vi "Get Contained Libraries.vi"(8 "error in":errorcluster, 10 "lib data in[]":T1[](array[typedef]), 11 "library in":refnum<vi>) -> (0 "error out":errorcluster, 3 "lib data out[]":T1[](array[typedef]))   [LabVIEW 2021, in "Converter.lvlib"]
uses:
  Converter.lvlib
  TypeDefs/Library Data.ctl
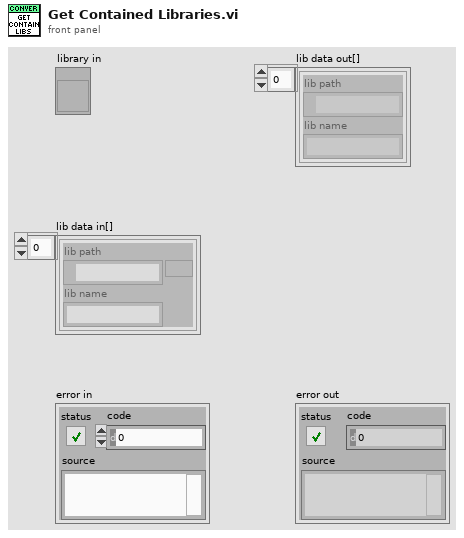
[diagram p1: front panel]
types:
  T1 = typedef "Converter.lvlib/Library Data.ctl" = cluster{"lib path":path, "lib name":string}
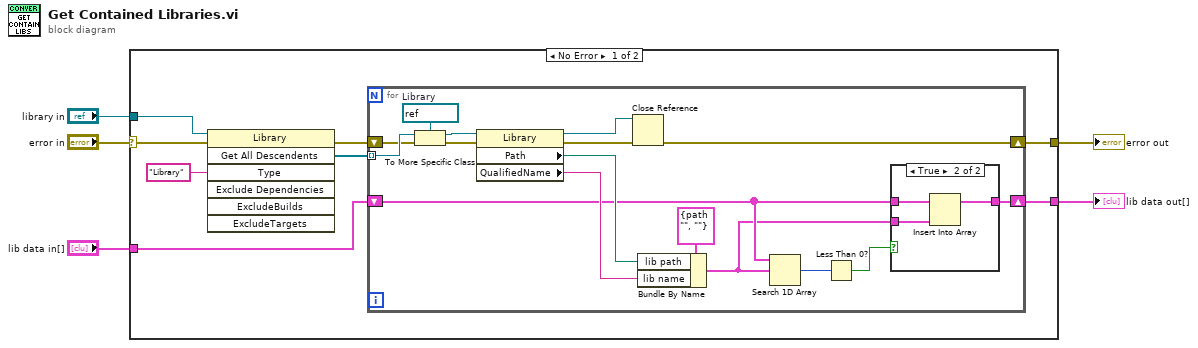
[diagram p0: block diagram]
diagram:
  n1 = case shown="No Error" "error in" {
    selector: "error in" -> [w13 w35]
    tunnel: [w6 w35] -> w5
    tunnel: "lib data in[]" -> [w12 w34]
    tunnel: [w11 w34] -> w2
    tunnel: "library in" -> [w8 _]
    frame No Error {
      n2 = invoke class="Library" method="Get All Descendents"(reference=w8, error in=w13, "Type"="Library") -> (error out=w10:errorcluster, "All Descendents"=w9:refnum<vi>[])  [unwired: 4 in, 5 out]
      n3 = for {
        tunnel: w9 -> [w29] mode=indexing
        shift-right: [w24] -> w11
        shift-left: w12 -> [w17]
        shift-right: [w14] -> w6
        shift-left: w10 -> [w27]
        w25 = refnum<vi> refnum  # Library
        n4 = To More Specific Class(target class=w25, reference=w29, error in=w27) -> (specific class reference=w28:refnum<vi>, error out=w26:errorcluster)
        n5 = property class="Library"(reference=w28, error in=w26) -> (reference out=w19:refnum<vi>, error out=w20:errorcluster, "Path"=w22:path, "QualifiedName"=w21:string)
        n6 = Close Reference(reference=w19, error in (no error)=w20) -> (error out=w14:errorcluster)
        n7 = Bundle By Name(cluster=T1 {"lib path"=path "", "lib name"=""}, "lib path"=w22, "lib name"=w21) -> (w16:T1)
        n8 = Search 1D Array(1D array=w17, element=w16) -> (index of element=w18:i32)  [unwired: 1 in]
        n9 = Less Than 0?(x=w18) -> (x < 0?=w15:bool)
        n10 = case shown="True" w15 {
          tunnel: [w30 w33] -> w24
          tunnel: w17 -> [w30 w32]
          tunnel: w16 -> [_ w31]
          frame False {
          }
          frame True {
            n11 = Insert Into Array(array=w32, new element=w31) -> (w33:T1[])  [unwired: 1 in]
          }
        }
      }
    }
    frame Error {
    }
  }
  "error out" <- w5
  "lib data out[]" <- w2
